vi "toggle.vi"(1 "Input":bool) -> (0 "Output":bool)   [LabVIEW 2014]
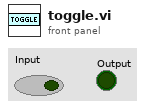
[diagram p1: front panel]
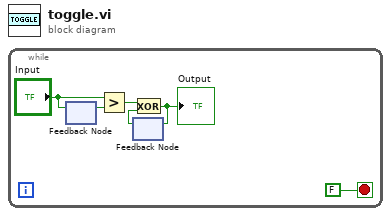
[diagram p0: block diagram]
diagram:
  n1 = while {
    stop <- FALSE stop-if-true
    n2 = feedback #1() -> (w5:bool)  [unwired: 1 in]
    n3 = feedback-in #1("Input") -> ()
    n4 = Greater?(x="Input", y=w5) -> (0:w4:bool)
    n5 = feedback #2() -> (w2:bool)  [unwired: 1 in]
    n6 = Exclusive Or(1:w2, 2:w4) -> (0:w3:bool)
    "Output" <- w3
    n7 = feedback-in #2(w3) -> ()
  }
